vi "Main2-backup.vi"() -> ()   [LabVIEW 2014]
uses:
  Control/Control_process.ctl
  Program Files (x86)/National Instruments/LabVIEW 2018/instr.lib/OSICS 1.1.0/OSICS_LIB.lvlib
  <vilib>/Utility/file.llb/Write Delimited Spreadsheet (string).vi
panel:
  out "error IO":errorcluster
  out "Test_pts_array":dbl[](array[numeric])
  out "WL_now":dbl
  in  "stop":bool
  in  "WL_delay(ms)":u32=800
  in  "VISA_PWM":refnum<visa-resource-name> caption="Power Meter"
  in  "VISA_TLS":refnum<visa-resource-name>="GPIB::10::INSTR" caption="Light Source"
  in  "PM_delay(ms)":i32=100
  out "Ref dbm":dbl caption="Ref (dBm)"
  in  "WL_Set":dbl=1310.0 caption="Wavelength"
  out "pow_read":dbl caption="Pow"
  in  "WL_step":dbl=1.0 caption="Step(nm)"
  out "WL_Peak":dbl caption="Peak"
  in  "WL_End":dbl=1350.0 caption="End(nm)"
  in  "WL_Start":dbl=1260.0 caption="Start(nm)"
  in  "Link Button":bool
  in  "Unit(dB:T)":bool
  in  "Read Button":bool
  in  "Ref Button":bool
  in  "Ref_spec Button":bool
  out "REF?":bool caption="Ref. 1pt"
  out "testing?":bool caption="Bussy"
  out "link?":bool caption="Online"
  out "Msg":string
  in  "Sweep Button":bool
  out "pow_chart":dbl(graph)
  # "Equip."
  # "SWEEP"
  # "READ"
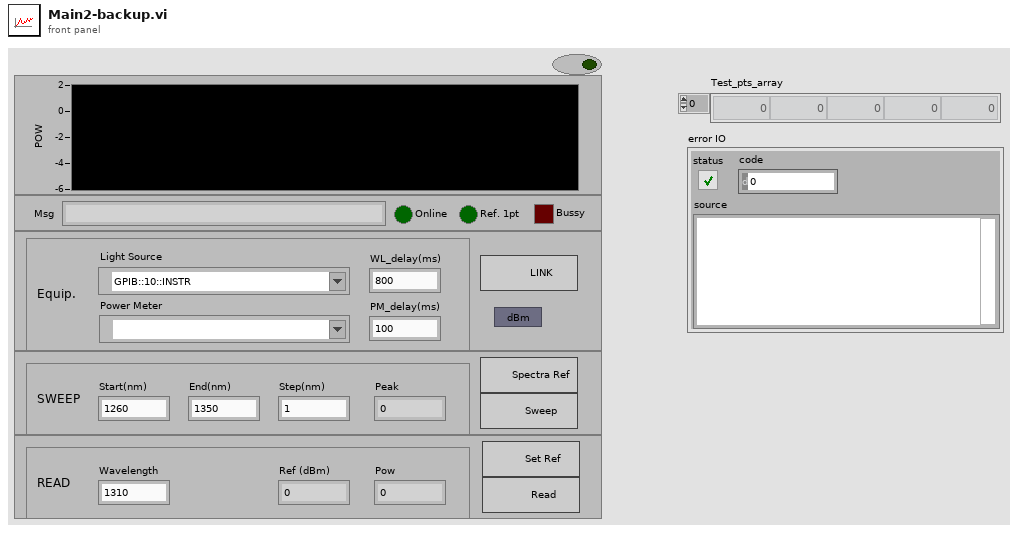
[diagram p1: front panel]
types:
  T1 = typedef "Control_process.ctl" = enum16{"init", "link", "reference", "reference2", "wave_chng", "lockpanel", "single", "sweep", "log_res", "quit"}
  T2 = enum8{"Enabled", "Disabled", "Disabled and Grayed Out"}
  T3 = cluster{"Laser State":bool, "WL/F Value":dbl, "Power (dBm/mW)":dbl, "Power Limit":bool}
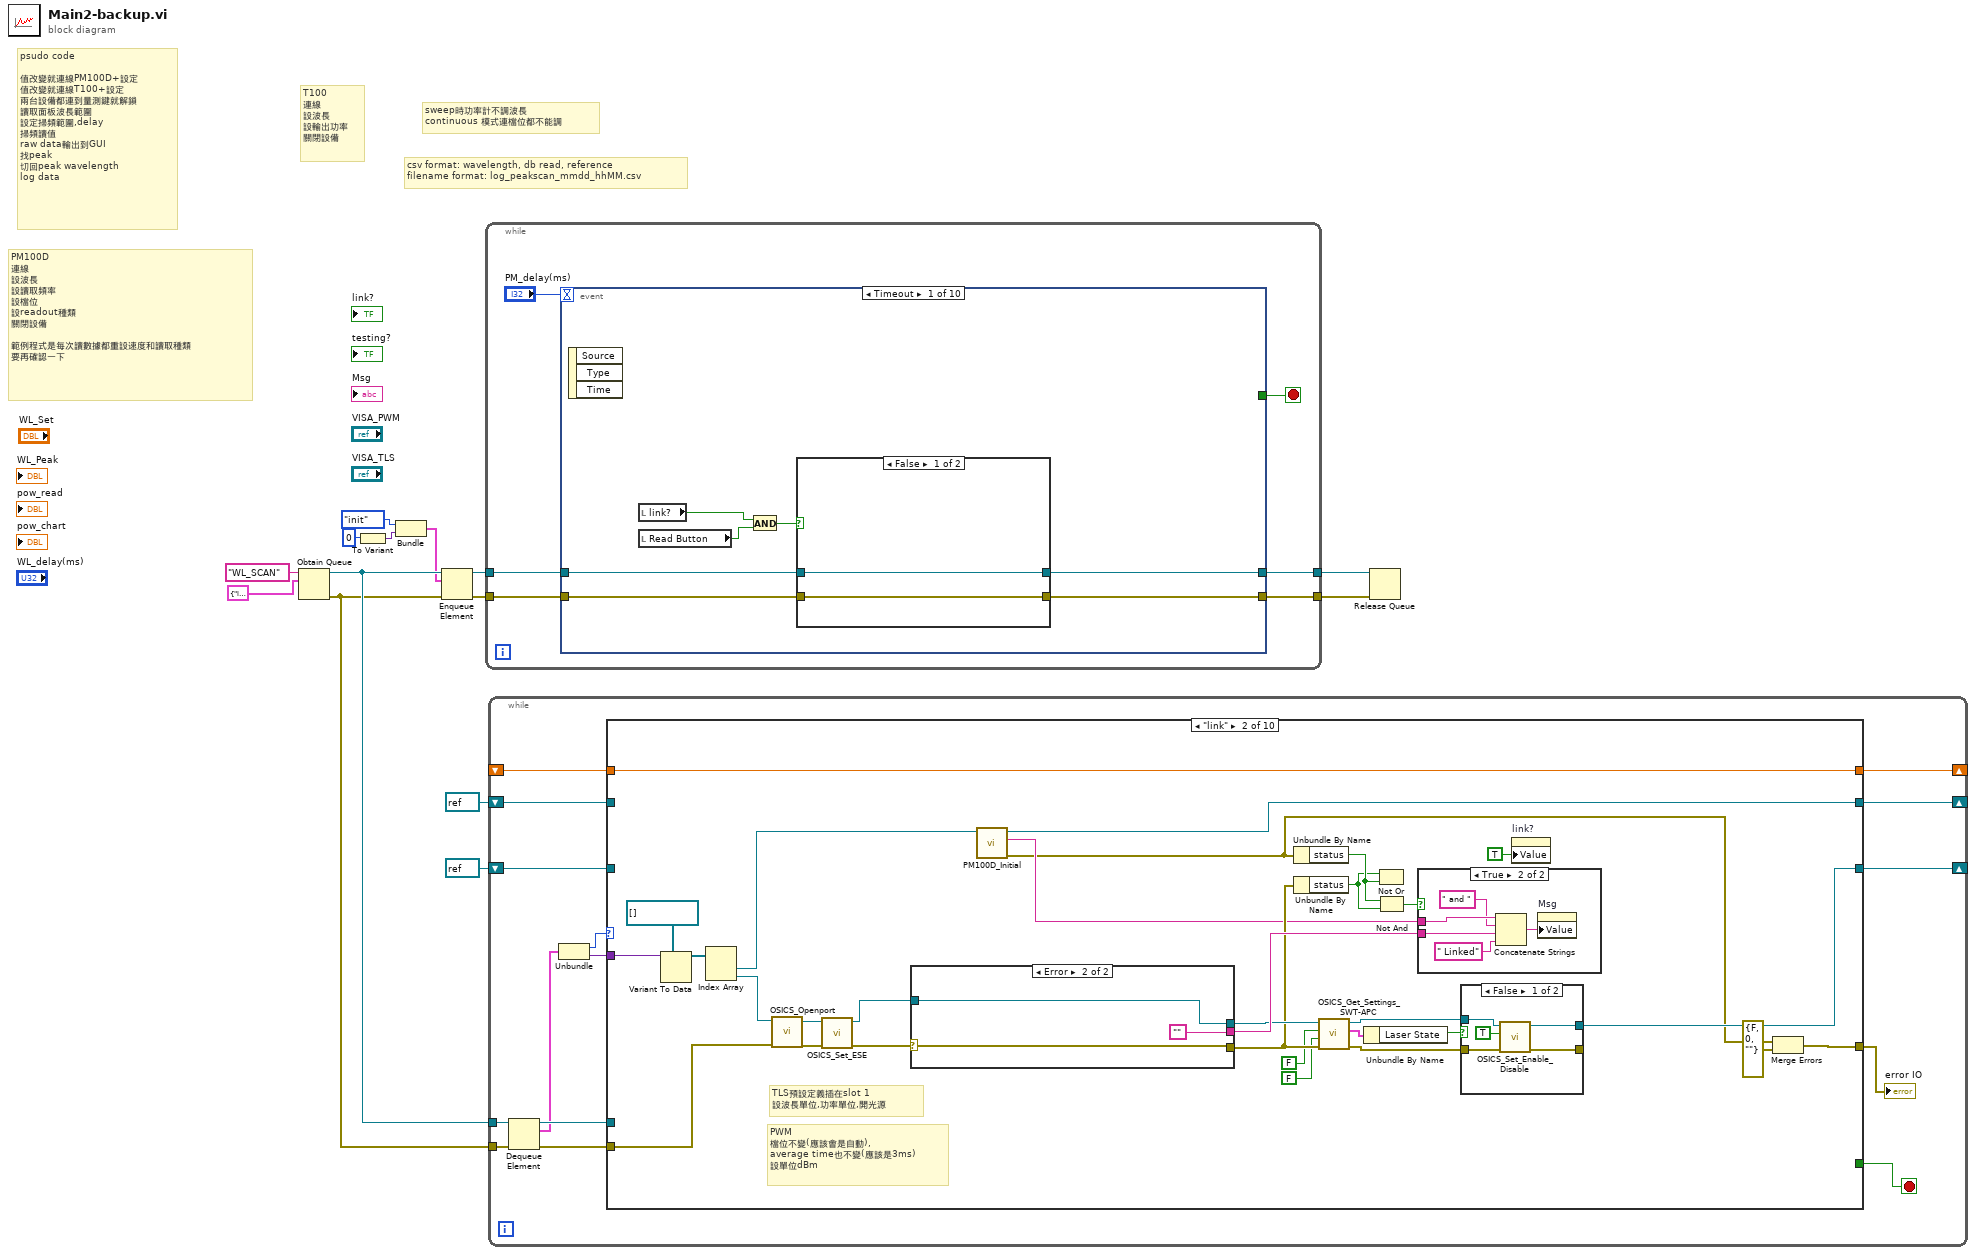
[diagram p0: block diagram]
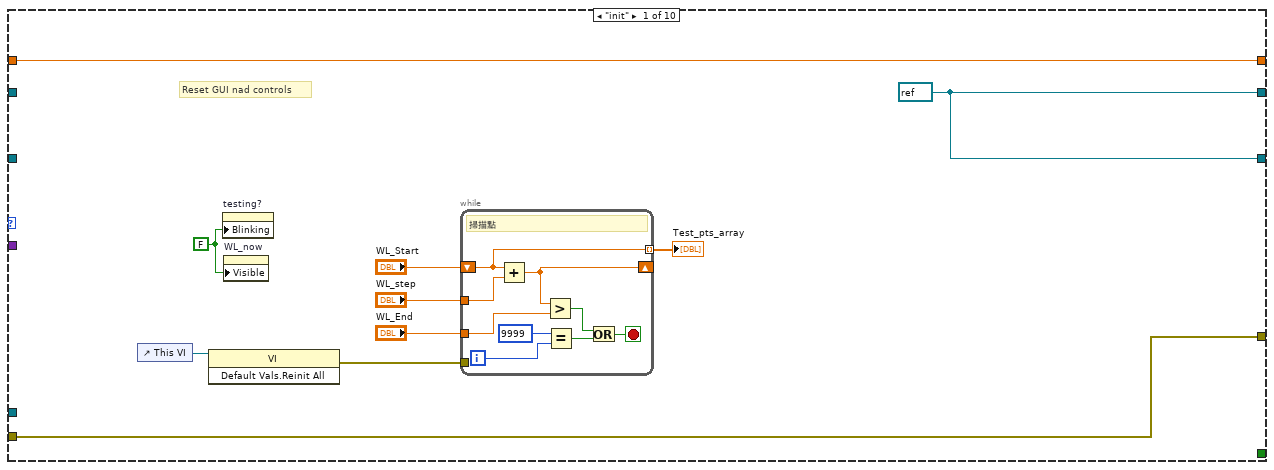
[diagram p2: hidden frame]
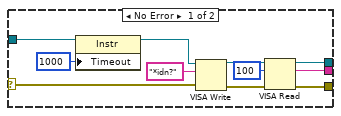
[diagram p3: hidden frame]
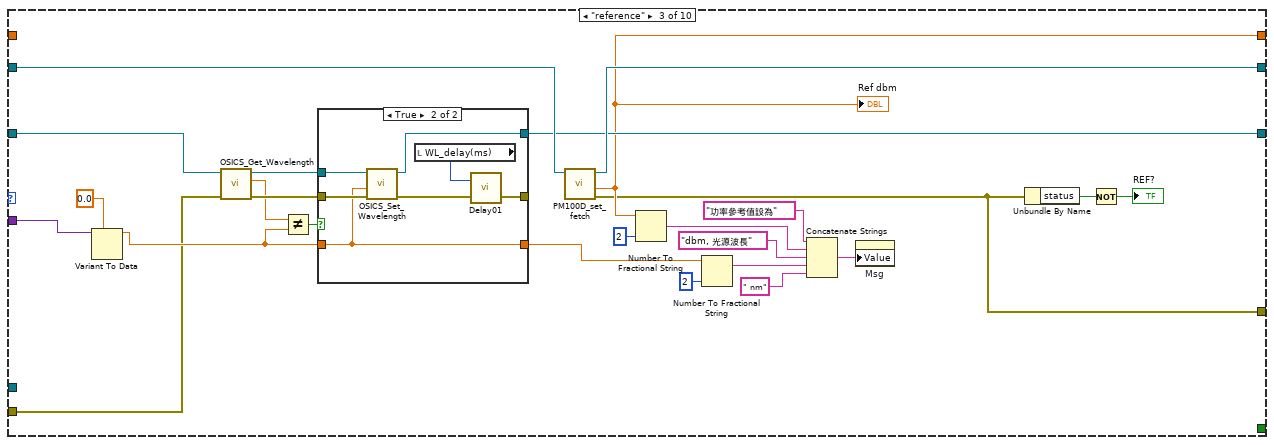
[diagram p6: hidden frame]
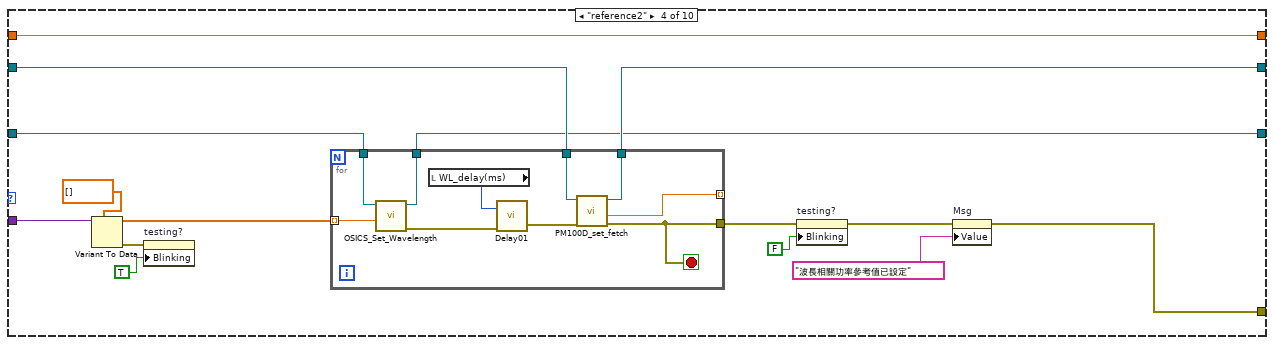
[diagram p8: hidden frame]
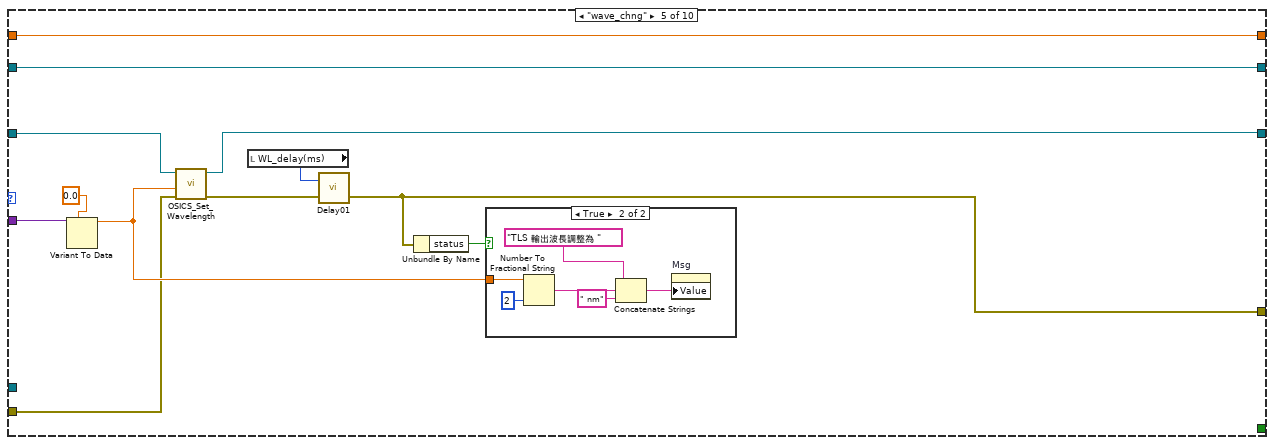
[diagram p9: hidden frame]
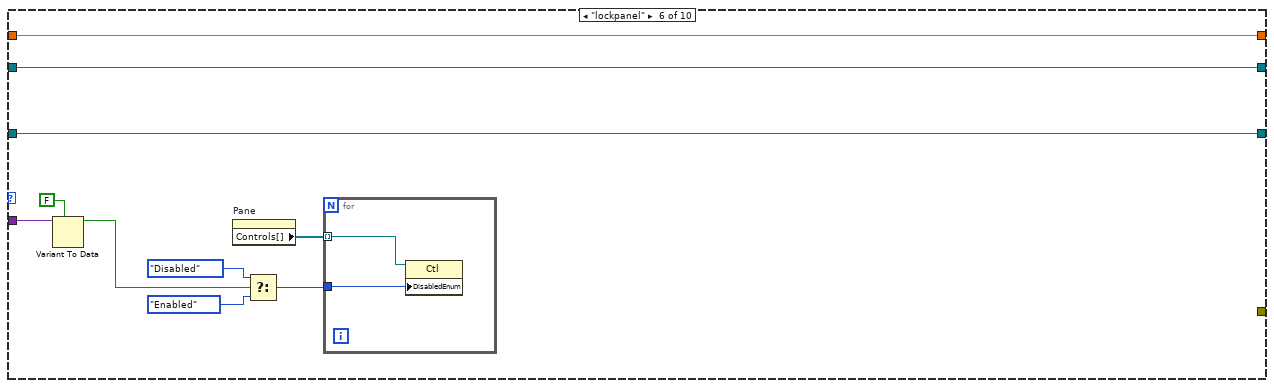
[diagram p11: hidden frame]
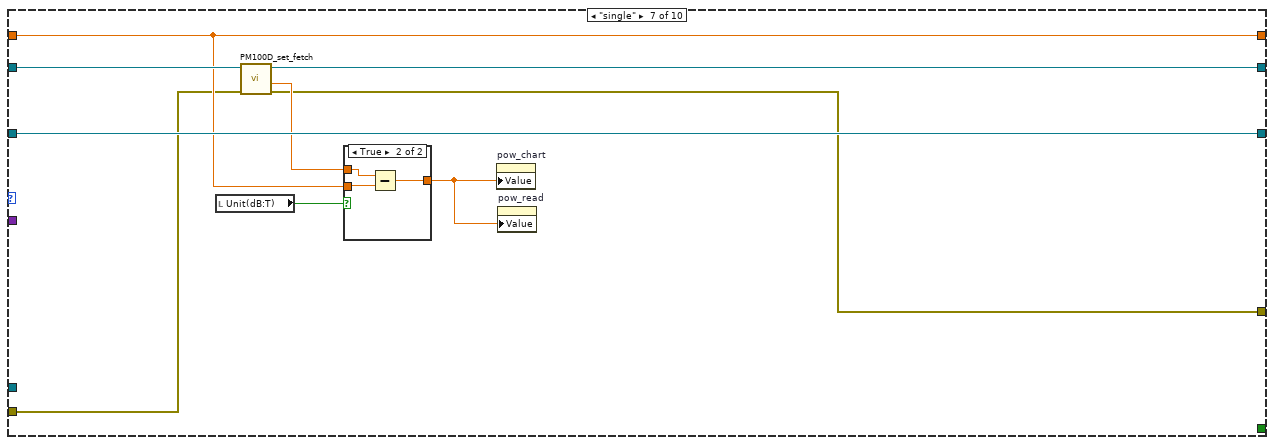
[diagram p12: hidden frame]
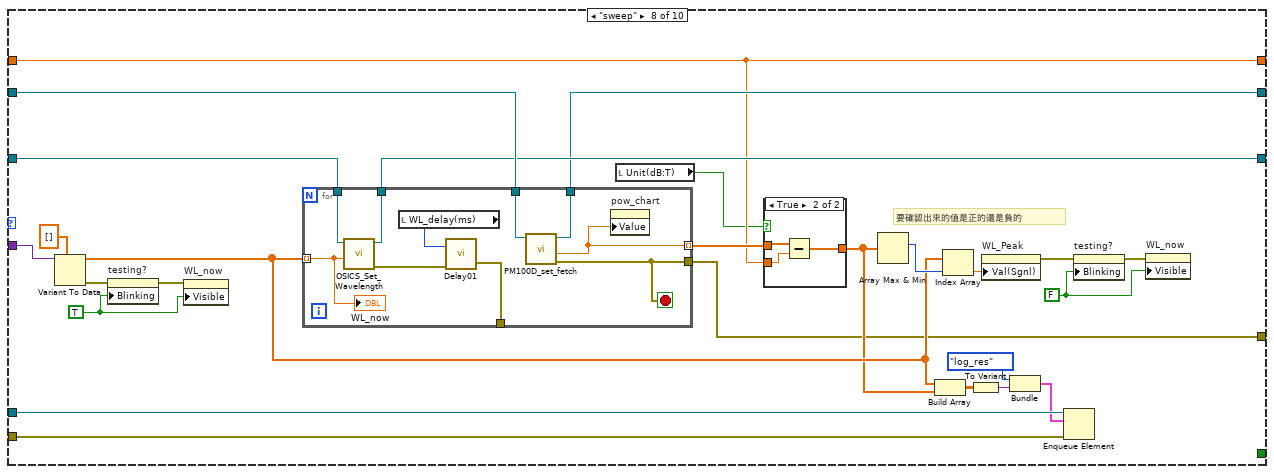
[diagram p14: hidden frame]
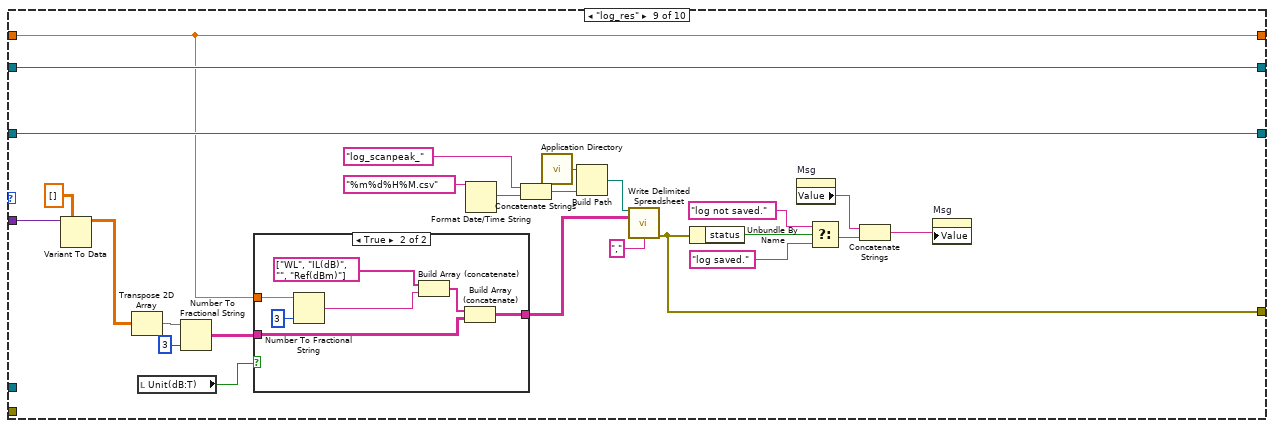
[diagram p16: hidden frame]
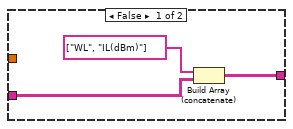
[diagram p17: hidden frame]
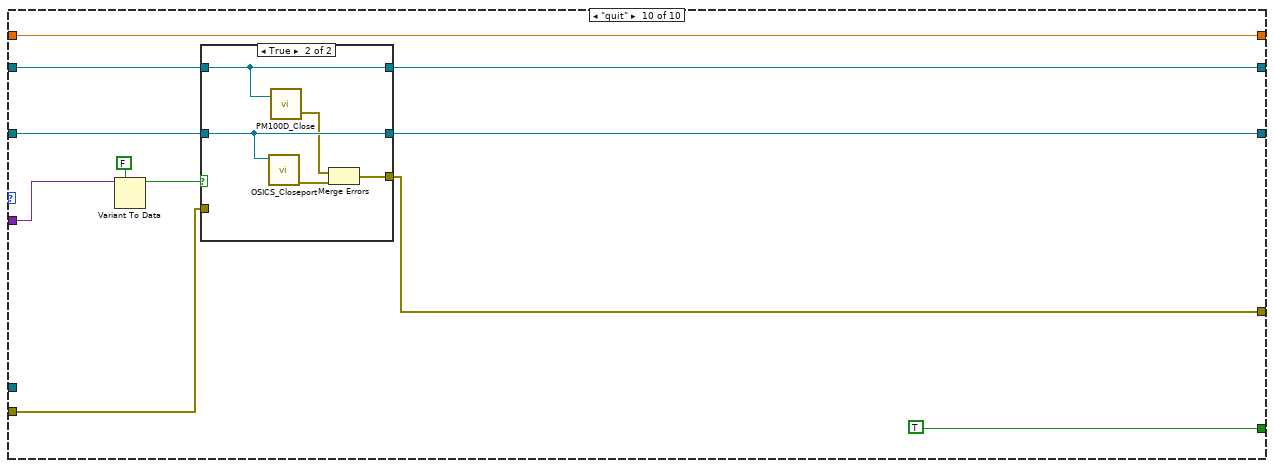
[diagram p18: hidden frame]
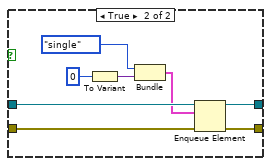
[diagram p20: hidden frame]
diagram:
  # "csv format: wavelength, db read, reference\nfilename format: log_peakscan_mmdd_hhMM.csv"
  # "sweep時功率計不調波長\ncontinuous 模式連檔位都不能調"
  # "T100\n連線\n設波長\n設輸出功率\n關閉設備"
  # "PM100D\n連線\n設波長\n設讀取頻率\n設檔位\n設readout種類\n關閉設備\n\n範例程式是每次讀數據都重設速度和讀取種類\n要再確認一下"
  # "psudo code\n\n值改變就連線PM100D+設定\n值改變就連線T100+設定\n兩台設備都連到量測鍵就解鎖\n讀取面板波長範圍\n設定掃頻範圍,delay\n掃頻讀值\nraw data輸出到GUI\n找peak\n切回peak wavelength\nlog data"
  n1 = Obtain Queue(name (unnamed)="WL_SCAN", element data type=cluster{"Proc":T1, variant} {"Proc"=enum."init", variant}) -> (queue out=w13:refnum<queue>, error out=w1:errorcluster)  [unwired: 3 in, 1 out]
  n2 = To Variant(anything=0) -> (Variant=w6:variant)
  n3 = Bundle("Proc"=Control_process."init", "Variant"=w6) -> (w4:cluster{"Proc":T1, "Variant":variant})  [unwired: 1 in]
  n4 = Enqueue Element(queue=w13, element=w4, error in (no error)=w1) -> (queue out=w9:refnum<queue>, error out=w8:errorcluster)  [unwired: 1 in, 1 out]
  n5 = while {
    tunnel: w9 -> [w18]
    tunnel: w8 -> [w19]
    tunnel: [w17] -> w12
    tunnel: [w16] -> w11
    stop <- w20 stop-if-true
    n6 = event shown="[0] Timeout" {
      selector: _ -> [_ _ _ _ _ _ _ _ _ _]
      dyn-events: _ -> [_ _ _ _ _ _ _ _ _ _]
      timeout: "PM_delay(ms)" -> [_ _ _ _ _ _ _ _ _ _]
      tunnel: [_ _ _ _ _ _ _ _ _ TRUE] -> w20
      tunnel: w19 -> [w26 w39 w47 w69 w83 w99 w130 w140 w168 w190]
      tunnel: w18 -> [w27 w40 w48 w70 w84 w100 w126 w142 w171 w188]
      tunnel: [w25 w40 w46 w70 w82 w98 w125 w141 w170 w187] -> w17
      tunnel: [w24 w39 w45 w69 w81 w97 w130 w139 w169 w189] -> w16
      event Timeout {
        n7 = event-data() -> ()  [unwired: 1 in, 3 out]
        n8 = local read "link?"() -> (w21:bool)
        n9 = local read "Read Button"() -> (w22:bool)
        n10 = And(x=w21, y=w22) -> (x .and. y?=w23:bool)
        n11 = case shown="False" w23 {
          tunnel: w27 -> [w29 w37]
          tunnel: w26 -> [w28 w36]
          tunnel: [w29 w35] -> w25
          tunnel: [w28 w34] -> w24
          frame False {
          }
          frame True {
            n12 = To Variant(anything=0) -> (Variant=w33:variant)
            n13 = Bundle("Proc"=Control_process."single", "Variant"=w33) -> (w31:cluster{"Proc":T1, "Variant":variant})  [unwired: 1 in]
            n14 = Enqueue Element(queue=w37, element=w31, error in (no error)=w36) -> (queue out=w35:refnum<queue>, error out=w34:errorcluster)  [unwired: 1 in, 1 out]
          }
        }
      }
      event "Unit(dB:T)": Value Change {
        # "這個事件會卡有紀錄參考值才能把單位轉dB"
        n15 = event-data() -> ()  [unwired: 1 in, 6 out]
        n16 = local read "REF?"() -> (w38:bool)
        n17 = case shown="False" w38 {
          frame False {
            n18 = property on="Unit(dB:T)" class="Bool (strict)"("Value"=FALSE ("Unit")) -> ()  [unwired: 2 in, 2 out]
            n19 = property on="Msg" class="Str"("Value"="Err: 參考值未設定" ("Msg")) -> ()  [unwired: 2 in, 2 out]
          }
          frame True {
          }
        }
      }
      event "Link Button": Value Change {
        n20 = event-data() -> ()  [unwired: 1 in, 1 out]
        n21 = local read "VISA_PWM"() -> (w43:refnum<visa-resource-name>)
        n22 = local read "VISA_TLS"() -> (w44:refnum<visa-resource-name>)
        n23 = Empty String/Path?(string/path=w44) -> (empty?=w50:bool)
        n24 = Empty String/Path?(string/path=w43) -> (empty?=w51:bool)
        n25 = Not Or(1:w50, 2:w51) -> (0:w49:bool)
        n26 = case shown="True" w49 {
          tunnel: w48 -> [w54 w64]
          tunnel: w47 -> [w53 w63]
          tunnel: [w54 w62] -> w46
          tunnel: [w53 w61] -> w45
          tunnel: w43 -> [_ w58]
          tunnel: w44 -> [_ w57]
          frame False {
            n27 = property on="Msg" class="Str"("Value"="Err: 未選擇儀器位址" ("Msg")) -> ()  [unwired: 2 in, 2 out]
          }
          frame True {
            n28 = Build Array(w58, w57) -> (w56:refnum<visa-resource-name>[])
            n29 = To Variant(anything=w56) -> (Variant=w55:variant)
            n30 = Bundle("Proc"=Control_process."link", "Variant"=w55) -> (w59:cluster{"Proc":T1, "Variant":variant})  [unwired: 1 in]
            n31 = Enqueue Element(queue=w64, element=w59, error in (no error)=w63) -> (queue out=w62:refnum<queue>, error out=w61:errorcluster)  [unwired: 1 in, 1 out]
          }
        }
      }
      event "WL_Start", "WL_End", "WL_step": Value Change {
        n32 = event-data() -> ()  [unwired: 1 in, 6 out]
        n33 = local read "WL_Start"() -> (w66:dbl)
        n34 = local read "WL_step"() -> (w68:dbl)
        n35 = local read "WL_End"() -> (w67:dbl)
        n36 = while {
          tunnel: w68 -> [w74]
          tunnel: w67 -> [w73]
          shift-right: [w75] -> _
          shift-left: w66 -> [w76]
          tunnel: [w76] -> w65 mode=indexing
          i -> [w72]
          stop <- w71 stop-if-true
          # "掃描點"
          n37 = Add(x=w76, y=w74) -> (x+y=w75:dbl)
          n38 = Greater?(x=w75, y=w73) -> (0:w78:bool)
          n39 = Equal?(x=9999, y=w72) -> (x = y?=w77:bool)
          n40 = Or(x=w78, y=w77) -> (x .or. y?=w71:bool)
        }
        n41 = local write "Test_pts_array"(w65) -> ()
      }
      event "Ref Button": Value Change {
        n42 = event-data() -> ()  [unwired: 1 in, 6 out]
        n43 = local read "link?"() -> (w80:bool)
        n44 = case shown="True" w80 {
          tunnel: w84 -> [w87 w95]
          tunnel: w83 -> [w86 w94]
          tunnel: [w87 w93] -> w82
          tunnel: [w86 w92] -> w81
          frame False {
            n45 = property on="Msg" class="Str"("Value"="Err: 設備未連結" ("Msg")) -> ()  [unwired: 2 in, 2 out]
          }
          frame True {
            n46 = local read "WL_Set"() -> (w88:dbl)
            n47 = To Variant(anything=w88) -> (Variant=w91:variant)
            n48 = Bundle("Proc"=Control_process."reference", "Variant"=w91) -> (w89:cluster{"Proc":T1, "Variant":variant})  [unwired: 1 in]
            n49 = Enqueue Element(queue=w95, element=w89, error in (no error)=w94) -> (queue out=w93:refnum<queue>, error out=w92:errorcluster)  [unwired: 1 in, 1 out]
          }
        }
      }
      event "Ref_spec Button": Value Change {
        n50 = event-data() -> ()  [unwired: 1 in, 6 out]
        n51 = local read "link?"() -> (w96:bool)
        n52 = case shown="True" w96 {
          tunnel: w100 -> [w103 w111]
          tunnel: w99 -> [w102 w110]
          tunnel: [w103 w107] -> w98
          tunnel: [w102 w104] -> w97
          frame False {
            n53 = property on="Msg" class="Str"("Value"="Err: 設備未連結" ("Msg")) -> ()  [unwired: 2 in, 2 out]
          }
          frame True {
            n54 = To Variant(anything=TRUE) -> (Variant=w117:variant)
            n55 = Bundle("Proc"=Control_process."lockpanel", "Variant"=w117) -> (w119:cluster{"Proc":T1, "Variant":variant})  [unwired: 1 in]
            n56 = local read "WL_Set"() -> (w120:dbl)
            n57 = Enqueue Element(queue=w111, element=w119, error in (no error)=w110) -> (queue out=w105:refnum<queue>, error out=w109:errorcluster)  [unwired: 1 in, 1 out]
            n58 = To Variant(anything=w120) -> (Variant=w123:variant)
            n59 = Bundle("Proc"=Control_process."reference", "Variant"=w123) -> (w121:cluster{"Proc":T1, "Variant":variant})  [unwired: 1 in]
            n60 = Enqueue Element(queue=w105, element=w121, error in (no error)=w109) -> (queue out=w106:refnum<queue>, error out=w108:errorcluster)  [unwired: 1 in, 1 out]
            n61 = To Variant(anything=FALSE) -> (Variant=w114:variant)
            n62 = Bundle("Proc"=Control_process."lockpanel", "Variant"=w114) -> (w112:cluster{"Proc":T1, "Variant":variant})  [unwired: 1 in]
            n63 = Enqueue Element(queue=w106, element=w112, error in (no error)=w108) -> (queue out=w107:refnum<queue>, error out=w104:errorcluster)  [unwired: 1 in, 1 out]
          }
        }
      }
      event "Read Button": Value Change {
        n64 = event-data() -> ()  [unwired: 1 in, 6 out]
        n65 = local read "link?"() -> (w128:bool)
        n66 = And(x=w128, y="Read Button") -> (x .and. y?=w127:bool)
        n67 = case shown="True" w127 {
          selector: w127 -> [w135 w136]
          tunnel: w126 -> [w133 w137]
          tunnel: [w132 w137] -> w125
          tunnel: [FALSE ("Blinking") w136] -> w124
          frame False {
            n68 = property on="Read Button" class="Bool (strict)"("Value"=w135) -> ()  [unwired: 2 in, 2 out]
            n69 = property on="Msg" class="Str"("Value"="Err: 設備未連結" ("Msg")) -> ()  [unwired: 2 in, 2 out]
            n70 = Flush Queue(queue=w133) -> (queue out=w132:refnum<queue>)  [unwired: 1 in, 2 out]
          }
          frame True {
          }
        }
        n71 = property on="testing?" class="Bool (strict)"("Blinking"=w124) -> ()  [unwired: 2 in, 2 out]
      }
      event "Sweep Button": Value Change {
        n72 = event-data() -> ()  [unwired: 1 in, 1 out]
        n73 = local read "link?"() -> (w138:bool)
        n74 = case shown="True" w138 {
          tunnel: w142 -> [w145 w149]
          tunnel: [w145 w155] -> w141
          tunnel: w140 -> [w144 w153]
          tunnel: [w144 w150] -> w139
          frame False {
            n75 = property on="Msg" class="Str"("Value"="Err: 設備未連結" ("Msg")) -> ()  [unwired: 2 in, 2 out]
          }
          frame True {
            n76 = To Variant(anything=TRUE) -> (Variant=w161:variant)
            n77 = Bundle("Proc"=Control_process."lockpanel", "Variant"=w161) -> (w162:cluster{"Proc":T1, "Variant":variant})  [unwired: 1 in]
            n78 = local read "Test_pts_array"() -> (w146:dbl[])
            n79 = Enqueue Element(queue=w149, element=w162, error in (no error)=w153) -> (queue out=w148:refnum<queue>, error out=w152:errorcluster)  [unwired: 1 in, 1 out]
            n80 = To Variant(anything=w146) -> (Variant=w165:variant)
            n81 = Bundle("Proc"=Control_process."sweep", "Variant"=w165) -> (w164:cluster{"Proc":T1, "Variant":variant})  [unwired: 1 in]
            n82 = Enqueue Element(queue=w148, element=w164, error in (no error)=w152) -> (queue out=w147:refnum<queue>, error out=w151:errorcluster)  [unwired: 1 in, 1 out]
            n83 = To Variant(anything=FALSE) -> (Variant=w158:variant)
            n84 = Bundle("Proc"=Control_process."lockpanel", "Variant"=w158) -> (w157:cluster{"Proc":T1, "Variant":variant})  [unwired: 1 in]
            n85 = Enqueue Element(queue=w147, element=w157, error in (no error)=w151) -> (queue out=w155:refnum<queue>, error out=w150:errorcluster)  [unwired: 1 in, 1 out]
            n86 = property on="Msg" class="Str"("Value"="波長掃描中......" ("Msg")) -> ()  [unwired: 2 in, 2 out]
          }
        }
      }
      event "WL_Set", "WL_Peak": Value Change {
        n87 = event-data() -> ("NewVal"=w172:dbl)  [unwired: 1 in]
        n88 = local read "link?"() -> (w167:bool)
        n89 = case shown="True" w167 {
          tunnel: w172 -> [_ w181]
          tunnel: w171 -> [w174 w179]
          tunnel: [w174 w178] -> w170
          tunnel: [w173 w177] -> w169
          tunnel: w168 -> [w173 w176]
          frame False {
          }
          frame True {
            n90 = To Variant(anything=w181) -> (Variant=w182:variant)
            n91 = Bundle("Proc"=Control_process."wave_chng", "Variant"=w182) -> (w175:cluster{"Proc":T1, "Variant":variant})  [unwired: 1 in]
            n92 = Enqueue Element(queue=w179, element=w175, error in (no error)=w176) -> (queue out=w178:refnum<queue>, error out=w177:errorcluster)  [unwired: 1 in, 1 out]
          }
        }
      }
      event "stop": Value Change {
        n93 = event-data() -> ()  [unwired: 1 in, 6 out]
        n94 = local read "link?"() -> (w183:bool)
        n95 = To Variant(anything=w183) -> (Variant=w185:variant)
        n96 = Bundle("Proc"=Control_process."quit", "Variant"=w185) -> (w184:cluster{"Proc":T1, "Variant":variant})  [unwired: 1 in]
        n97 = Enqueue Element At Opposite End(queue=w188, element=w184, error in (no error)=w190) -> (queue out=w187:refnum<queue>, error out=w189:errorcluster)  [unwired: 1 in, 1 out]
      }
    }
  }
  n98 = while {
    tunnel: w13 -> [w206]
    shift-right: [w196] -> _
    shift-left: refnum<visa-resource-name> refnum ("instrument handle out") -> [w200]
    shift-right: [w199] -> _
    shift-left: refnum<visa-resource-name> refnum ("VISA OUT") -> [w198]
    shift-right: [w195] -> _
    shift-left: _ -> [w194]
    tunnel: w1 -> [w192]
    stop <- w197 stop-if-true
    n99 = Dequeue Element(queue=w206, error in (no error)=w192) -> (queue out=w205:refnum<queue>, element=w203:cluster{"Proc":T1, variant}, error out=w204:errorcluster)  [unwired: 1 in, 1 out]
    n100 = Unbundle(w203) -> ("Proc"=w202:T1, w201:variant)
    n101 = case shown="\"link\"" w202 {
      tunnel: w205 -> [_ _ _ _ _ _ _ w402 _ _]
      tunnel: w204 -> [w213 w229 w285 _ w342 _ w372 w401 _ w461]
      tunnel: w201 -> [_ w255 w304 w331 w351 w362 _ w409 w448 w465]
      tunnel: w200 -> [_ _ w306 w326 w346 w368 w380 w410 w433 w468]
      tunnel: [w216 w239 w303 w324 w352 w367 w379 w408 w444 w466] -> w199
      tunnel: w198 -> [_ _ w301 w327 w353 w367 w379 w407 w444 w470]
      tunnel: [_ _ _ _ _ _ _ _ _ TRUE] -> w197
      tunnel: [w216 w231 w305 w325 w346 w368 w378 w396 w433 w467] -> w196
      tunnel: [w213 w235 w284 w317 w343 _ w373 w391 w427 w460] -> w193
      tunnel: [w214 w236 w286 w328 w344 w369 w376 w394 w426 w462] -> w195
      tunnel: w194 -> [w214 w236 _ w328 w344 w369 w376 w394 w426 w462]
      frame "init" {
        w212 = FALSE ("Blinking")
        w216 = refnum<visa-resource-name> refnum ("instrument handle out")
        # "Reset GUI nad controls"
        n102 = control-ref of="This VI"() -> (w215:refnum<vi>)
        n103 = invoke class="VI" method="Default Vals.Reinit All"(reference=w215) -> (error out=w207:errorcluster)  [unwired: 2 in, 2 out]
        n104 = property on="testing?" class="Bool (strict)"("Blinking"=w212) -> ()  [unwired: 2 in, 2 out]
        n105 = property on="WL_now" class="DigNum (strict)"("Visible"=w212) -> ()  [unwired: 2 in, 2 out]
        n106 = while {
          tunnel: "WL_step" -> [w220]
          tunnel: "WL_End" -> [w219]
          shift-right: [w221] -> _
          shift-left: "WL_Start" -> [w222]
          tunnel: [w222] -> w208 mode=indexing
          tunnel: w207 -> [_]
          i -> [w218]
          stop <- w217 stop-if-true
          # "掃描點"
          n107 = Add(x=w222, y=w220) -> (x+y=w221:dbl)
          n108 = Greater?(x=w221, y=w219) -> (0:w224:bool)
          n109 = Equal?(x=9999, y=w218) -> (x = y?=w223:bool)
          n110 = Or(x=w224, y=w223) -> (x .or. y?=w217:bool)
        }
        "Test_pts_array" <- w208
      }
      frame "link" {
        # "TLS預設定義插在slot 1\n設波長單位,功率單位,開光源"
        # "PWM\n檔位不變(應該會是自動), \naverage time也不變(應該是3ms)\n設單位dBm"
        n111 = Variant To Data(type=refnum<visa-resource-name>[] [], Variant=w255) -> (data=w254:refnum<visa-resource-name>[])  [unwired: 1 in, 1 out]
        n112 = Index Array(array=w254) -> (element #1=w232:refnum<visa-resource-name>, element #2=w252:refnum<visa-resource-name>)  [unwired: 2 in]
        n113 = call "OSICS_Openport.vi"("error in"=w229, "VISA IN"=w252) -> ("error out"=w253:errorcluster, "VISA OUT"=w251:refnum<visa-resource-name>)  [unwired: 8 in]
        n114 = call "OSICS_Set_ESE.vi"("error in (no error)"=w253, "VISA resource name"=w251) -> ("error out"=w228:errorcluster, "VISA resource name out"=w250:refnum<visa-resource-name>)  [unwired: 8 in]
        n115 = case shown="Error" w228 {
          selector: w228 -> [w256 w269]
          tunnel: w250 -> [w260 w268]
          tunnel: [w259 ""] -> w249
          tunnel: [w258 w268] -> w247
          tunnel: [w257 w269] -> w244
          frame No Error {
            n116 = property class="Instr"(reference=w260, "Timeout"=u32 1000 ("General Settings:Timeout Value")) -> (reference out=w265:refnum<visa-resource-name>)  [unwired: 1 in, 1 out]
            n117 = VISA Write(VISA resource name=w265, write buffer="*idn?", error in (no error)=w256) -> (VISA resource name out=w263:refnum<visa-resource-name>, error out=w261:errorcluster)  [unwired: 1 out]
            n118 = VISA Read(VISA resource name=w263, byte count=u32 100, error in (no error)=w261) -> (VISA resource name out=w258:refnum<visa-resource-name>, read buffer=w259:string, error out=w257:errorcluster)  [unwired: 1 out]
          }
          frame Error {
          }
        }
        n119 = call "PM100D_Initial.vi"("VISA in"=w232) -> ("error out"=w230:errorcluster, "IDN String"=w233:string, "VISA out"=w231:refnum<visa-resource-name>)  [unwired: 3 in, 1 out]
        n120 = Unbundle By Name(w230) -> ("status"=w238:bool)
        n121 = Unbundle By Name(w244) -> ("status"=w237:bool)
        n122 = call "OSICS_Get_Settings_SWT-APC.vi"("error in"=w244, "Power Unit(dBm/mW)"=FALSE, "WL/F unit (nm/GHz)"=FALSE, "VISA IN"=w247) -> ("error out"=w240:errorcluster, "Laser Settings (Cluster)"=w246:T3, "VISA OUT"=w241:refnum<visa-resource-name>)  [unwired: 5 in]
        n123 = Unbundle By Name(w246) -> ("Laser State"=w245:bool)
        n124 = Not Or(1:w238, 2:w237) -> ()  [unwired: 1 out]
        n125 = Not And(1:w237, 2:w238) -> (0:w248:bool)
        n126 = case shown="True" w248 {
          tunnel: w249 -> [_ w281]
          tunnel: w233 -> [_ w280]
          frame False {
          }
          frame True {
            n127 = Concatenate Strings(w280, " and " ("string"), w281, " Linked" ("string")) -> (w278:string)
            n128 = property on="Msg" class="Str"("Value"=w278) -> ()  [unwired: 2 in, 2 out]
          }
        }
        n129 = case shown="False" w245 {
          tunnel: w241 -> [w273 w276]
          tunnel: w240 -> [w272 w275]
          tunnel: [w271 w276] -> w239
          tunnel: [w270 w275] -> _
          frame False {
            n130 = call "OSICS_Set_Enable_Disable.vi"("error in"=w272, "Laser State (False:DISABLED)"=TRUE, "VISA IN"=w273) -> ("error out"=w270:errorcluster, "VISA OUT"=w271:refnum<visa-resource-name>)  [unwired: 6 in, 1 out]
          }
          frame True {
          }
        }
        n131 = property on="link?" class="Bool (strict)"("Value"=TRUE ("link?")) -> ()  [unwired: 2 in, 2 out]
        n132 = Merge Errors(w230, errorcluster {"status"=FALSE, "code"=0, "source"=""} ("error in")) -> (w235:errorcluster)
      }
      frame "reference" {
        n133 = Variant To Data(type=0.0, Variant=w304) -> (data=w287:dbl)  [unwired: 1 in, 1 out]
        n134 = call "OSICS_Get_Wavelength.vi"("error in"=w285, "VISA IN"=w301) -> ("error out"=w300:errorcluster, "WL/Frequency Value"=w298:dbl, "VISA OUT"=w302:refnum<visa-resource-name>)  [unwired: 6 in, 1 out]
        n135 = Not Equal?(x=w298, y=w287) -> (x != y?=w299:bool)
        n136 = case shown="True" w299 {
          tunnel: [w308 w314] -> _
          tunnel: [w309 w313] -> w303
          tunnel: w302 -> [w309 w312]
          tunnel: w300 -> [w308 w311]
          tunnel: w287 -> [w307 w310]
          tunnel: [w307 w310] -> w289
          frame False {
          }
          frame True {
            n137 = call "OSICS_Set_Wavelength.vi"("error in"=w311, "WL/Frequency Value"=w310, "VISA IN"=w312) -> ("error out"=w316:errorcluster, "VISA OUT"=w313:refnum<visa-resource-name>)  [unwired: 6 in, 1 out]
            n138 = local read "WL_delay(ms)"() -> (w315:u32)
            n139 = call "Delay01.vi"("error in"=w316, "ms delay"=w315) -> ("error out"=w314:errorcluster)  [unwired: 1 in]
          }
        }
        n140 = call "PM100D_set_fetch.vi"("VISA in"=w306) -> ("error out"=w284:errorcluster, "Readout value"=w286:dbl, "VISA out"=w305:refnum<visa-resource-name>)  [unwired: 6 in, 2 out]
        "Ref dbm" <- w286
        n141 = Number To Fractional String(number=w286, precision (6)=i16 2) -> (F-format string=w291:string)  [unwired: 2 in]
        n142 = Number To Fractional String(number=w289, precision (6)=i16 2) -> (F-format string=w295:string)  [unwired: 2 in]
        n143 = Concatenate Strings("功率參考值設為" ("string"), w291, "dbm, 光源波長" ("string"), w295, " nm" ("string")) -> (w294:string)
        n144 = property on="Msg" class="Str"("Value"=w294) -> ()  [unwired: 2 in, 2 out]
        n145 = Unbundle By Name(w284) -> ("status"=w283:bool)
        n146 = Not(x=w283) -> (.not. x?=→"REF?":bool)
      }
      frame "reference2" {
        n147 = Variant To Data(type=dbl[] [], Variant=w331) -> (data=w329:dbl[], error out=w320:errorcluster)  [unwired: 1 in]
        n148 = property on="testing?" class="Bool (strict)"(error in=w320, "Blinking"=TRUE) -> ()  [unwired: 1 in, 2 out]
        n149 = for {
          tunnel: w326 -> [w341]
          tunnel: [w340] -> w325
          tunnel: [w337] -> w324
          tunnel: w327 -> [w336]
          tunnel: [w333] -> w319
          tunnel: [w335] -> _ mode=indexing
          tunnel: w329 -> [w334] mode=indexing
          stop <- w333 stop-if-true
          n150 = call "OSICS_Set_Wavelength.vi"("WL/Frequency Value"=w334, "VISA IN"=w336) -> ("error out"=w339:errorcluster, "VISA OUT"=w337:refnum<visa-resource-name>)  [unwired: 7 in, 1 out]
          n151 = local read "WL_delay(ms)"() -> (w332:u32)
          n152 = call "Delay01.vi"("error in"=w339, "ms delay"=w332) -> ("error out"=w338:errorcluster)  [unwired: 1 in]
          n153 = call "PM100D_set_fetch.vi"("error in"=w338, "VISA in"=w341) -> ("error out"=w333:errorcluster, "Readout value"=w335:dbl, "VISA out"=w340:refnum<visa-resource-name>)  [unwired: 5 in, 2 out]
        }
        n154 = property on="testing?" class="Bool (strict)"(error in=w319, "Blinking"=FALSE) -> (error out=w318:errorcluster)  [unwired: 1 in, 1 out]
        n155 = property on="Msg" class="Str"(error in=w318, "Value"="波長相關功率參考值已設定" ("string")) -> (error out=w317:errorcluster)  [unwired: 1 in, 1 out]
      }
      frame "wave_chng" {
        n156 = Variant To Data(type=0.0, Variant=w351) -> (data=w345:dbl)  [unwired: 1 in, 1 out]
        n157 = call "OSICS_Set_Wavelength.vi"("error in"=w342, "WL/Frequency Value"=w345, "VISA IN"=w353) -> ("error out"=w349:errorcluster, "VISA OUT"=w352:refnum<visa-resource-name>)  [unwired: 6 in, 1 out]
        n158 = local read "WL_delay(ms)"() -> (w347:u32)
        n159 = call "Delay01.vi"("error in"=w349, "ms delay"=w347) -> ("error out"=w343:errorcluster)  [unwired: 1 in]
        n160 = Unbundle By Name(w343) -> ("status"=w348:bool)
        n161 = case shown="True" w348 {
          tunnel: w345 -> [_ w356]
          frame False {
          }
          frame True {
            n162 = Number To Fractional String(number=w356, precision (6)=i16 2) -> (F-format string=w355:string)  [unwired: 2 in]
            n163 = Concatenate Strings("TLS 輸出波長調整為 " ("Msg"), w355, " nm" ("string")) -> (w359:string)
            n164 = property on="Msg" class="Str"("Value"=w359) -> ()  [unwired: 2 in, 2 out]
          }
        }
      }
      frame "lockpanel" {
        n165 = Variant To Data(type=FALSE, Variant=w362) -> (data=w360:bool)  [unwired: 1 in, 1 out]
        n166 = property on="Pane" class="Pane"() -> ("Controls[]"=w366:refnum<vi>[])  [unwired: 2 in, 2 out]
        n167 = Select(t=T2."Disabled" ("Disabled"), s=w360, f=T2."Enabled" ("Disabled")) -> (s? t:f=w365:T2)
        n168 = for {
          tunnel: w366 -> [w371] mode=indexing
          tunnel: w365 -> [w370]
          n169 = property on="Property Node" class="Ctl"(reference=w371, "DisabledEnum"=w370) -> ()  [unwired: 1 in, 2 out]
        }
      }
      frame "single" {
        n170 = local read "Unit(dB:T)"() -> (w374:bool)
        n171 = call "PM100D_set_fetch.vi"("error in"=w372, "VISA in"=w380) -> ("error out"=w373:errorcluster, "Readout value"=w377:dbl, "VISA out"=w378:refnum<visa-resource-name>)  [unwired: 5 in, 2 out]
        n172 = case shown="True" w374 {
          tunnel: w377 -> [w381 w384]
          tunnel: w376 -> [_ w383]
          tunnel: [w381 w382] -> w375
          frame False {
          }
          frame True {
            n173 = Subtract(x=w384, y=w383) -> (x-y=w382:dbl)
          }
        }
        n174 = property on="pow_chart" class="WFChart (strict)"("Value"=w375) -> ()  [unwired: 2 in, 2 out]
        n175 = property on="pow_read" class="DigNum (strict)"("Value"=w375) -> ()  [unwired: 2 in, 2 out]
      }
      frame "sweep" {
        w385 = TRUE ("Blinking")
        w386 = FALSE ("Blinking")
        # "要確認出來的值是正的還是負的"
        n176 = Variant To Data(type=dbl[] [], Variant=w409) -> (data=w403:dbl[], error out=w390:errorcluster)  [unwired: 1 in]
        n177 = property on="testing?" class="Bool (strict)"(error in=w390, "Blinking"=w385) -> (error out=w388:errorcluster)  [unwired: 1 in, 1 out]
        n178 = property on="WL_now" class="DigNum (strict)"(error in=w388, "Visible"=w385) -> ()  [unwired: 1 in, 2 out]
        n179 = for {
          tunnel: w410 -> [w424]
          tunnel: [w423] -> w396
          tunnel: [w420] -> w408
          tunnel: w407 -> [w419]
          tunnel: [w416] -> w391
          tunnel: [w418] -> w395 mode=indexing
          tunnel: w403 -> [w417] mode=indexing
          tunnel: [w415] -> _
          stop <- w416 stop-if-true
          n180 = call "OSICS_Set_Wavelength.vi"("WL/Frequency Value"=w417, "VISA IN"=w419) -> ("error out"=w422:errorcluster, "VISA OUT"=w420:refnum<visa-resource-name>)  [unwired: 7 in, 1 out]
          n181 = local read "WL_delay(ms)"() -> (w421:u32)
          n182 = call "Delay01.vi"("error in"=w422, "ms delay"=w421) -> ("error out"=w415:errorcluster)  [unwired: 1 in]
          n183 = call "PM100D_set_fetch.vi"("VISA in"=w424) -> ("error out"=w416:errorcluster, "Readout value"=w418:dbl, "VISA out"=w423:refnum<visa-resource-name>)  [unwired: 6 in, 2 out]
          n184 = property on="pow_chart" class="WFChart (strict)"("Value"=w418) -> ()  [unwired: 2 in, 2 out]
          "WL_now" <- w417
        }
        n185 = local read "Unit(dB:T)"() -> (w392:bool)
        n186 = case shown="True" w392 {
          tunnel: w395 -> [w411 w414]
          tunnel: w394 -> [_ w413]
          tunnel: [w411 w412] -> w393
          frame False {
          }
          frame True {
            n187 = Subtract(x=w414, y=w413) -> (x-y=w412:dbl[])
          }
        }
        n188 = Array Max & Min(array=w393) -> (max index (indices)=w405:i32)  [unwired: 3 out]
        n189 = Build Array(w403, w393) -> (w398:dbl[][])
        n190 = Index Array(array=w403, index=w405) -> (element=w404:dbl)
        n191 = To Variant(anything=w398) -> (Variant=w399:variant)
        n192 = property on="WL_Peak" class="DigNum (strict)"("Val(Sgnl)"=w404) -> (error out=w389:errorcluster)  [unwired: 2 in, 1 out]
        n193 = Bundle("Proc"=Control_process."log_res", "Variant"=w399) -> (w397:cluster{"Proc":T1, "Variant":variant})  [unwired: 1 in]
        n194 = Enqueue Element(queue=w402, element=w397, error in (no error)=w401) -> ()  [unwired: 1 in, 3 out]
        n195 = property on="testing?" class="Bool (strict)"(error in=w389, "Blinking"=w386) -> (error out=w387:errorcluster)  [unwired: 1 in, 1 out]
        n196 = property on="WL_now" class="DigNum (strict)"(error in=w387, "Visible"=w386) -> ()  [unwired: 1 in, 2 out]
      }
      frame "log_res" {
        n197 = Variant To Data(type=dbl[][] [] ("appended array"), Variant=w448) -> (data=w430:dbl[][])  [unwired: 1 in, 1 out]
        n198 = Transpose 2D Array(2D array=w430) -> (transposed array=w431:dbl[][])
        n199 = local read "Unit(dB:T)"() -> (w425:bool)
        n200 = Number To Fractional String(number=w431, precision (6)=i16 3) -> (F-format string=w429:string[][])  [unwired: 2 in]
        n201 = case shown="True" w425 {
          tunnel: w429 -> [w452 w459]
          tunnel: [w450 w458] -> w428
          tunnel: w426 -> [_ w455]
          frame False {
            n202 = Build Array (concatenate)(string[] ["WL", "IL(dBm)"], w452) -> (w450:string[][])
          }
          frame True {
            n203 = Number To Fractional String(number=w455, precision (6)=i16 3) -> (F-format string=w454:string)  [unwired: 2 in]
            n204 = Build Array (concatenate)(string[] ["WL", "IL(dB)", "", "Ref(dBm)"], w454) -> (w457:string[])
            n205 = Build Array (concatenate)(w457, w459) -> (w458:string[][])
          }
        }
        n206 = Format Date/Time String(time format string (%c)="%m%d%H%M.csv") -> (date/time string=w441:string)  [unwired: 2 in]
        n207 = Concatenate Strings("log_scanpeak_" ("string"), w441) -> (w440:string)
        n208 = call <vilib>:"Application Directory.vi"() -> ("Application Directory"=w446:path)
        n209 = Build Path(base path=w446, name or relative path=w440) -> (appended path=w445:path)
        n210 = call-poly <vilib>:"Write Delimited Spreadsheet.vi"("file path (dialog if empty)"=w445, "2D data"=w428, "delimiter (\\t)"="," ("delimiter (\\t)")) -> ("error out"=w427:errorcluster)  [unwired: 11 in, 1 out]
        n211 = Unbundle By Name(w427) -> ("status"=w439:bool)
        n212 = property on="Msg" class="Str"() -> ("Value"=w436:string)  [unwired: 2 in, 2 out]
        n213 = Select(t="log not saved.", s=w439, f="log saved.") -> (s? t:f=w437:string)
        n214 = Concatenate Strings(w436, w437) -> (w438:string)
        n215 = property on="Msg" class="Str"("Value"=w438) -> ()  [unwired: 2 in, 2 out]
      }
      frame "quit" {
        n216 = Variant To Data(type=FALSE, Variant=w465) -> (data=w463:bool)  [unwired: 1 in, 1 out]
        n217 = case shown="True" w463 {
          tunnel: w470 -> [w472 w477]
          tunnel: w468 -> [w473 w478]
          tunnel: [w473 w478] -> w467
          tunnel: [w472 w477] -> w466
          tunnel: w461 -> [w471 _]
          tunnel: [w471 w475] -> w460
          frame False {
          }
          frame True {
            n218 = call "OSICS_Closeport.vi"("VISA IN"=w477) -> ("error out"=w476:errorcluster)  [unwired: 10 in]
            n219 = call "PM100D_Close.vi"("VISA resource name"=w478) -> ("error out"=w474:errorcluster)  [unwired: 2 in]
            n220 = Merge Errors(w474, w476) -> (w475:errorcluster)
          }
        }
      }
    }
    "error IO" <- w193
  }
  n221 = Release Queue(queue=w12, error in (no error)=w11) -> ()  [unwired: 1 in, 3 out]
